vi "Disable SEN.vi"(8 "error in (no error)":errorcluster, 11 "SGDV_Ctrl_Class in":refnum<class "SGDV_Ctrl_Class.lvclass">) -> (0 "error out":errorcluster, 3 "SGDV_Ctrl_Class out":refnum<class "SGDV_Ctrl_Class.lvclass">)   [LabVIEW 2013, in "SGDV_Ctrl_v13_lib.lvlib" / "SGDV_Ctrl_Class.lvclass"]
uses:
  SGDV_Ctrl_Class.lvclass
  SGDV_Ctrl_Class.lvclass/SGDV_Ctrl_Class.ctl
  SGDV_Ctrl_v13_lib.lvlib
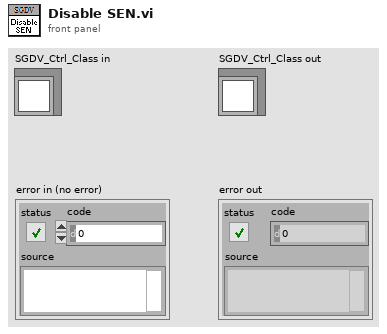
[diagram p1: front panel]
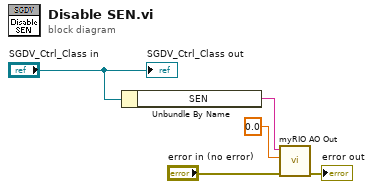
[diagram p0: block diagram]
diagram:
  n1 = Unbundle By Name("SGDV_Ctrl_Class in") -> ("SEN"=w3:tag)
  n2 = call "myRIO AO Out.vi"("error in (no error)"="error in (no error)", "Value"=0.0 ("A/AO0 (Pin 2)"), "Motor IO Refnum.SEN"=w3) -> ("error out"=→"error out":errorcluster)  [unwired: 8 in]
  "SGDV_Ctrl_Class out" <- "SGDV_Ctrl_Class in"
